vi "Test Process Wait For Lifecycle State While Clearing Does Not Time Out.vi"(8 "error in (no error)":errorcluster, 11 "Process Test In":refnum<class "Process Test.lvclass">) -> (0 "error out":errorcluster, 3 "Process Test Out":refnum<class "Process Test.lvclass">)   [LabVIEW 2020, in "Process Test.lvclass"]
uses:
  Process Test.lvclass
  C:/Program Files (x86)/National Instruments/LabVIEW 2020/vi.lib/Asteme/LUnit/Test Case.lvclass
  Framework/Process/Public/Lifecycle/Lifecycle State.ctl
  <vilib>/Asteme/LUnit/Test Case.lvclass/Test Case.ctl
  <vilib>/Asteme/LUnit/LUnit Assertion Result.lvclass/LUnit Assertion Result.ctl
  <vilib>/Asteme/LUnit/Palette/Fail.vi
  <vilib>/Asteme/LUnit/Palette/Pass.vi
  <vilib>/Asteme/LUnit/Set Assertion Type.vi
  <vilib>/Asteme/LUnit/Palette/Pass If.vi
  <vilib>/Asteme/LUnit/Add test result.vi
  <vilib>/Asteme/LUnit/LUnit Write Passed.vi
  <vilib>/Asteme/LUnit/LUnit Get Test Case.vi
  <vilib>/Asteme/LUnit/Assertion Result/LUnit Get Test Name.vi
  <vilib>/Asteme/LUnit/LUnit Write Message.vi
  <vilib>/Asteme/LUnit/LUnit Write Description.vi
  <vilib>/Asteme/LUnit/LUnit Write Assertion Type.vi
  <vilib>/Asteme/LUnit/Read Test Case Name.vi
  <vilib>/Asteme/LUnit/LUnit Assertion Result.lvclass
  Framework/Process/Process.lvclass
  <vilib>/Asteme/LUnit/Test Case.lvclass
  C:/Users/anton/Documents/GitHub/Triarc-Framework/source/Framework Test/Base Class Test/Base Test.lvclass
  C:/Users/anton/Documents/GitHub/Triarc-Framework/source/Framework Test/Process Test/Process Test.lvclass
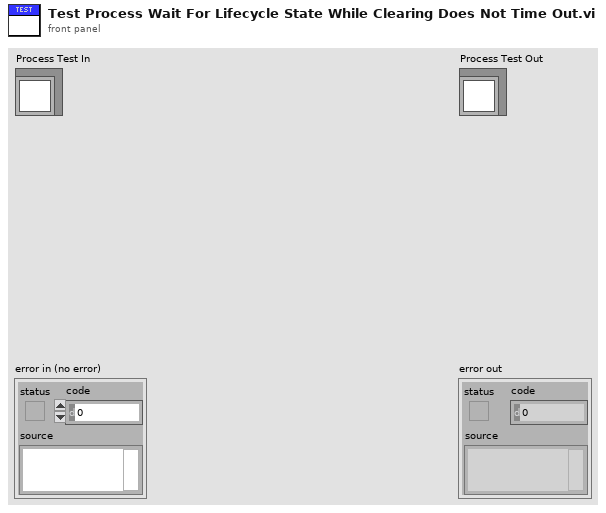
[diagram p1: front panel]
types:
  T1 = typedef "Process.lvclass/Lifecycle State.ctl" = enum16{"Uninitialized", "Initialized", "Started", "Running", "Stopped", "Finished"}
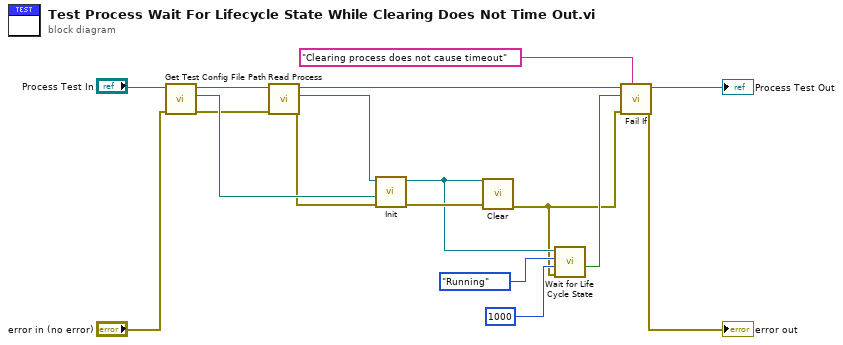
[diagram p0: block diagram]
diagram:
  n1 = call-dynamic "Get Test Config File Path.vi"("error in (no error)"="error in (no error)", "Base Class Test in"="Process Test In") -> ("error out"=w10:errorcluster, "Test config path"=w13:path, "Base Class Test out"=w15:refnum<class "Process Test.lvclass">)  [unwired: 7 in]
  n2 = call "Read Process.vi"("error in (no error)"=w10, "Process Test in"=w15) -> ("error out"=w11:errorcluster, "Process.lvclass"=w12:refnum<class "Process.lvclass">, "Process Test out"=w8:refnum<class "Process Test.lvclass">)  [unwired: 7 in]
  n3 = call-dynamic "Init.vi"("error in (no error)"=w11, "Config File Path"=w13, "Process In"=w12) -> ("error out"=w16:errorcluster, "Process Out"=w9:refnum<class "Process.lvclass">)  [unwired: 7 in]
  n4 = call-dynamic "Clear.vi"("error in (no error)"=w16, "Process In"=w9) -> ("error out"=w1:errorcluster)  [unwired: 9 in]
  n5 = call "Wait for Life Cycle State.vi"("error in (no error)"=w1, "timeout in ms (-1)"=1000, "Lifecycle State"=Lifecycle_State."Running", "Process In"=w9) -> ("timed out?"=w2:bool)  [unwired: 5 in, 2 out]
  n6 = call <vilib>:"Fail If.vi"("Description"="Clearing process does not cause timeout", "error in (no error)"=w1, "Fail?"=w2, "Test Case In"=w8) -> ("error out"=→"error out":errorcluster, "Test Case Out"=→"Process Test Out":refnum<class "Process Test.lvclass">)  [unwired: 6 in]
